vi "force sensor.vi"   [LabVIEW 2010, in "Rampage.lvrbt"]
uses:
  Rampage.lvrbt
  <vilib>/NXT/Block Support/NXT_InputPort.ctl
  <vilib>/NXT/Dual Mode Library/Display/drawNumber.vi
types:
  T1 = typedef "NXT_InputPort.ctl" = u8
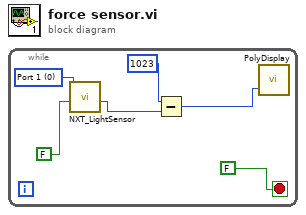
[diagram p0: block diagram]
diagram:
  n1 = while {
    stop <- FALSE stop-if-true
    w5 = T1 0 items=["Port 1", "Port 2", "Port 3", "Port 4"] ("Input (Port 3)")
    n2 = call <vilib>:"NXT_LightSensor.vi"("Floodlight"=FALSE, "Input (Port 3)"=w5) -> ("Raw Value"=w4:u16)  [unwired: 6 in, 3 out]
    n3 = Subtract(x=u16 1023, y=w4) -> (x-y=w2:u16)
    n4 = call-poly <vilib>:"PolyDisplay.vi"("number"=w2) -> ()  [unwired: 3 in, 1 out]
  }
